vi "Process.vi"(8 "error in":errorcluster, 11 "Example Instrument UI":refnum<class "Instrument.PPMS2 UI.lvclass">) -> (0 "error out":errorcluster, 3 "Example Instrument UI out":refnum<class "Instrument.PPMS2 UI.lvclass">)   [LabVIEW 2016, in "Instrument.PPMS2 UI.lvclass"]
doc: "---------------------------------------------------------------\nJKI State Machine Objects™\nhttp://jki.net/state-machine-objects/\nCopyright (C) 2005-2015, JKI <info@jki.net>\nALL RIGHTS RESERVEDJKI State Machine Objects (SMO) 1.0.0.5\nJKI - JKI\nCopyright (c) 2016, JKI"
uses:
  Instrument.PPMS2 UI.lvclass
  C:/Program Files (x86)/National Instruments/LabVIEW 2016/vi.lib/JKI/JKI SMO/SMO/SMO.lvclass
  C:/Program Files (x86)/National Instruments/LabVIEW 2016/vi.lib/JKI/JKI SMO/SMO.UI/SMO.UI.lvclass
  instrument.PPMS2/Typedefs/Magnet Status--PPMS2--ring.ctl
  instrument.PPMS2/Typedefs/Temperature Status--PPMS2--ring.ctl
  <vilib>/JKI/JKI SMO/SMO/Typedefs/Parent Call--Enum.ctl
  <userlib>/LevyLab/Levylab Instruments/SMOs/RemoteControl.STM/RemoteControl.STM.lvclass
  Instrument.PPMS2 UI.lvclass/Instrument.PPMS2 UI.ctl
  instrument.PPMS2/Typedefs/getAll--PPMS2--cluster.ctl
  <vilib>/JKI/JKI SMO/SMO.UI/SMO.UI.lvclass
  <userlib>/LevyLab/Levylab Instruments/SMOs/Instrument/Instrument.lvclass
  <vilib>/JKI/JKI SMO/SMO/SMO.lvclass
  instrument.PPMS2/instrument.PPMS2.lvclass
panel:
  in  "Angle":bool
  in  "Field":bool
  in  "Temperature":bool
  in  "Target Angle (°)":dbl=-0.00643419474363327 format="%_3g"
  in  "Target Field (Oe)":dbl=-0.00643419474363327 format="%_3g"
  in  "Target Temperature (K)":dbl=305.0156 format="%#_5g"
  out "Temperature Status":T1 items=["TemperatureUnknown"=0, "Stable"=1, "Tracking"=2, "Near"=5, "Chasing"=6, "Filling"=7, "Standby"=10, "Disabled"=13, "ImpedanceNotFunction"=14, "TempFailure"=15]
  out "Field Status":T2=1 items=["MagnetUnknown"=0, "StablePersistent"=1, "WarmingSwitch"=2, "CoolingSwitch"=3, "StableDriven"=4, "Iterating"=5, "Charging"=6, "Discharging"=7, "CurrentError"=8, "MagnetFailure"=15]
  out "Helium Level (%)":dbl=86.7
  out "Position (°)":dbl=90.002
  out "Field (Oe)":dbl=-0.00643419474363327 format="%_3g"
  out "Temperature(K)":dbl=305.0156 format="%#_5g"
  in  "update time (ms)":u32=200
  in  "STOP":bool
  # "PPMS 2 Monitor"
  # "SMO UI Template"
  # "For instructions on how to use the JKI State Machine Objects, examples and video tutorials, visit:\nhttp://jki.net/state-machine-objects/\n\nJKI State Machine Objects™\nhttp://jki.net/state-machine-objects/\nCopyright (C) 2005-2015, JKI <info@jki.net>\nALL RIGHTS RESERVED"
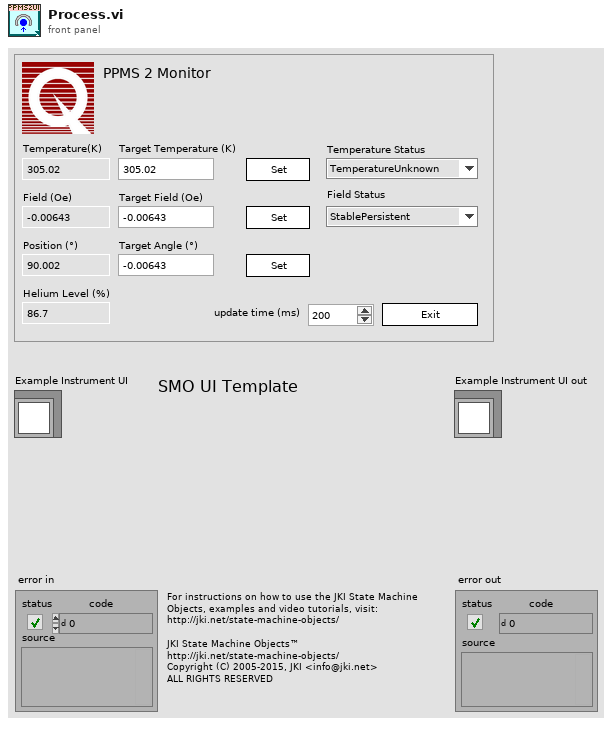
[diagram p1: front panel]
types:
  T1 = typedef "instrument.PPMS2.lvclass/Temperature Status--PPMS2--ring.ctl" = i32
  T2 = typedef "instrument.PPMS2.lvclass/Magnet Status--PPMS2--ring.ctl" = i32
  T3 = typedef "SMO.lvclass/Parent Call--Enum.ctl" = enum16{"Allows parent to run", "Does not request parent to run"}
  T4 = enum32{"invalid app kind", "Development System", "Run Time System", "Student Edition", "Embedded LabVIEW", "Evaluation", "Custom"}
  T5 = enum32{"Invalid", "Standard", "Closed", "Hidden", "Minimized", "Maximized"}
  T6 = typedef "instrument.PPMS2.lvclass/getAll--PPMS2--cluster.ctl" = cluster{"PPMS 2 Helium Level":dbl, "PPMS 2 Temperature":dbl, "PPMS 2 Temperature Status":T1, "PPMS 2 Magnetic Field":dbl, "PPMS 2 Magnet Status":T2, "PPMS 2 Position":dbl}
  T7 = cluster{"Core":cluster{"Current VI Reference":refnum<vi>, "Close Panel on Exit?":bool, "error":errorcluster}, "Self Reference":refnum<class "Instrument.PPMS2 UI.lvclass">, "Instrument":refnum<class "Instrument.lvclass">, "RC.STM":refnum<class "RemoteControl.STM.lvclass">, "getAll":variant, "getDisplay":variant, "config":variant}
  T8 = cluster{"Current VI Reference":refnum<vi>, "Close Panel on Exit?":bool, "error":errorcluster}
  T9 = typedef "SMO.lvclass/Protected Events.ctl" = cluster{"StopProcesses":refnum<user-event>, "AbortProcesses":refnum<user-event>, "Config Changed":refnum<user-event>, "Dependency":refnum<user-event>}
  T10 = typedef "Instrument.lvclass/PublicEvents--Cluster.ctl" = cluster{"MessageFromProcess":refnum<user-event>}
  T11 = typedef "Instrument.lvclass/Configuration--Cluster.ctl" = cluster{"Hardware":cluster{"Address":string, "Type":string, "COM Type":string}, "SMO":cluster{"VI Address":string, "Port":i32}, "DSC":cluster{"Process Name":string}}
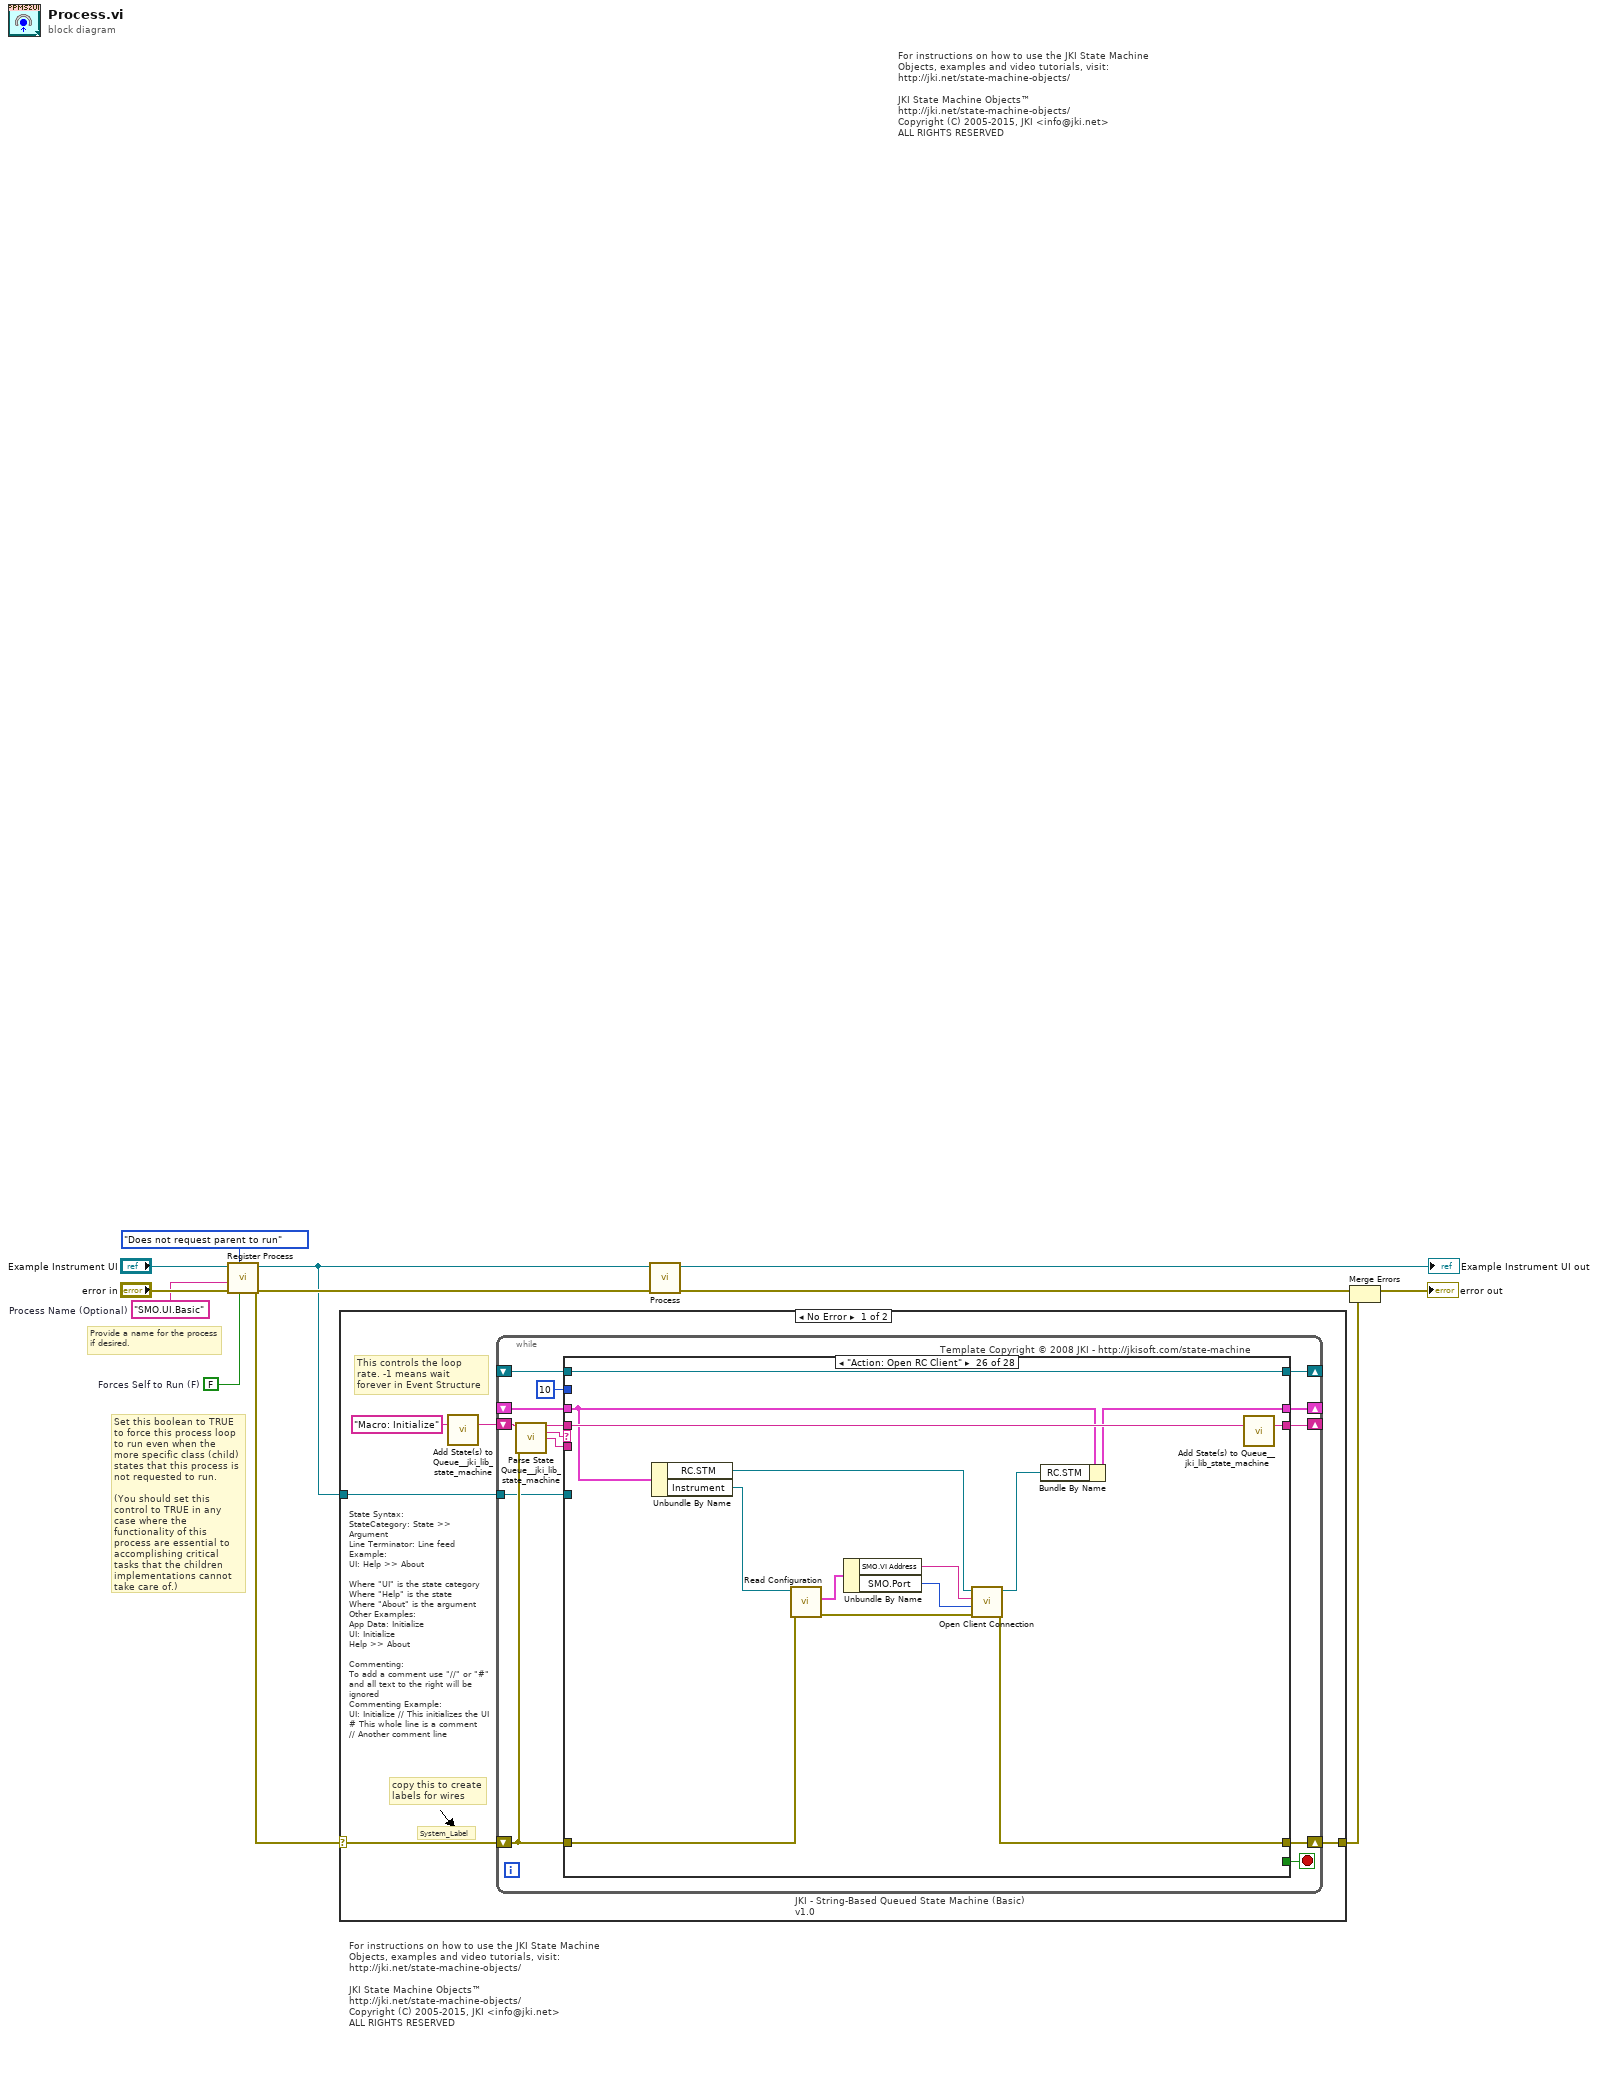
[diagram p0: block diagram]
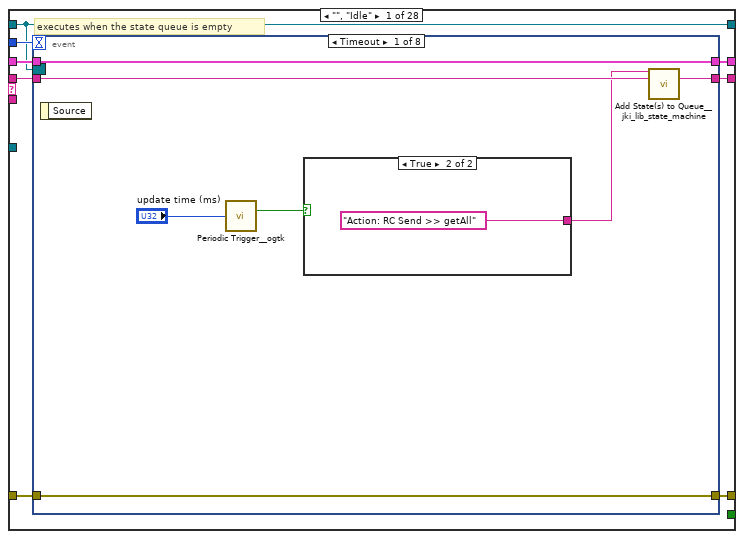
[diagram p2: hidden frame]
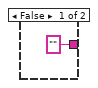
[diagram p3: hidden frame]
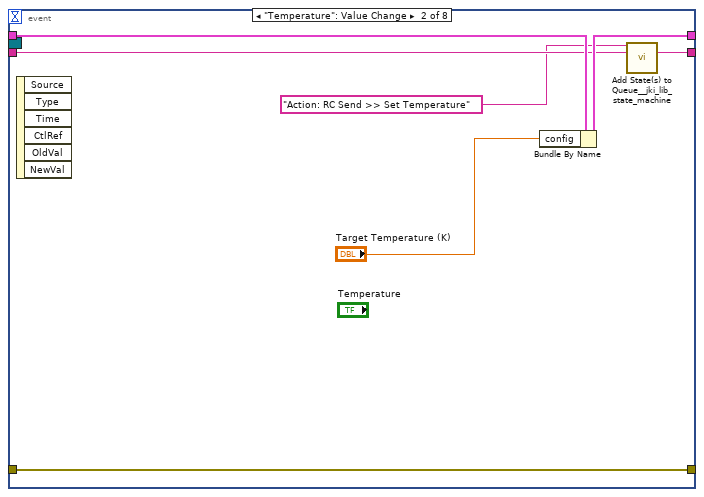
[diagram p4: hidden frame]
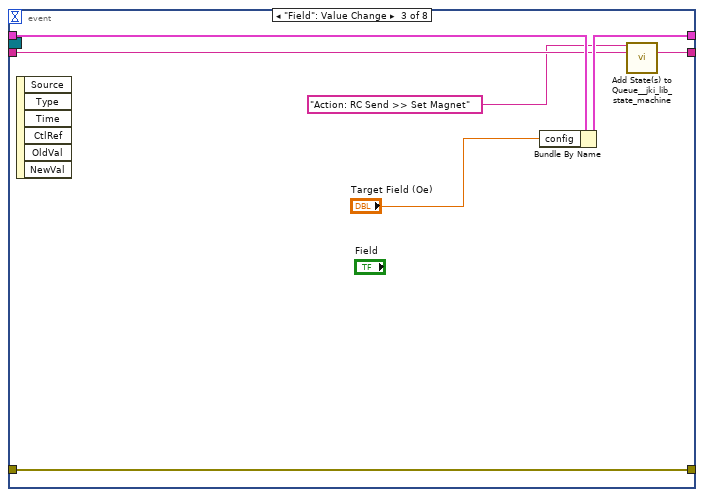
[diagram p5: hidden frame]
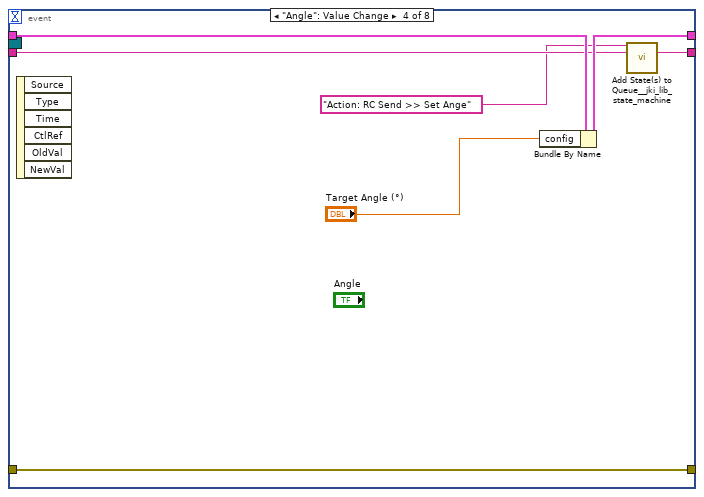
[diagram p6: hidden frame]
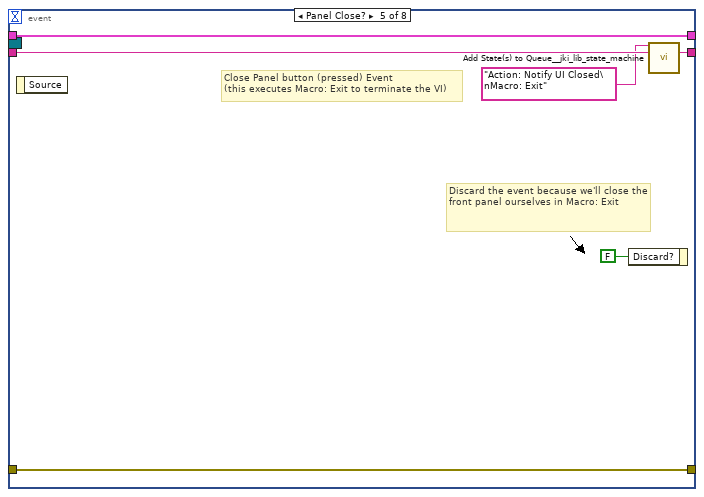
[diagram p7: hidden frame]
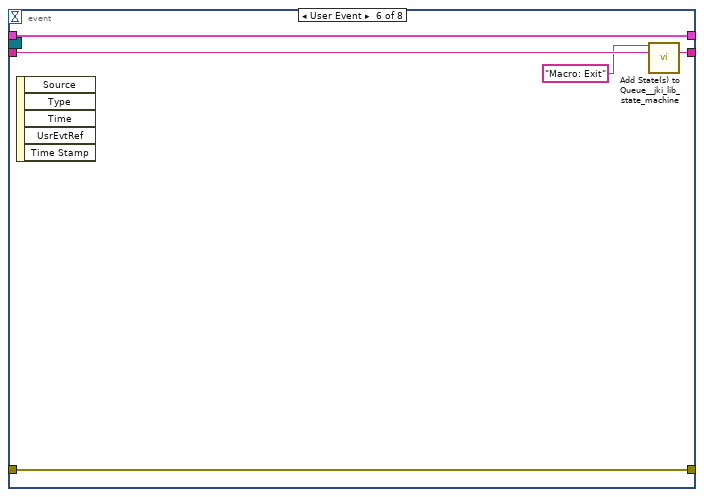
[diagram p8: hidden frame]
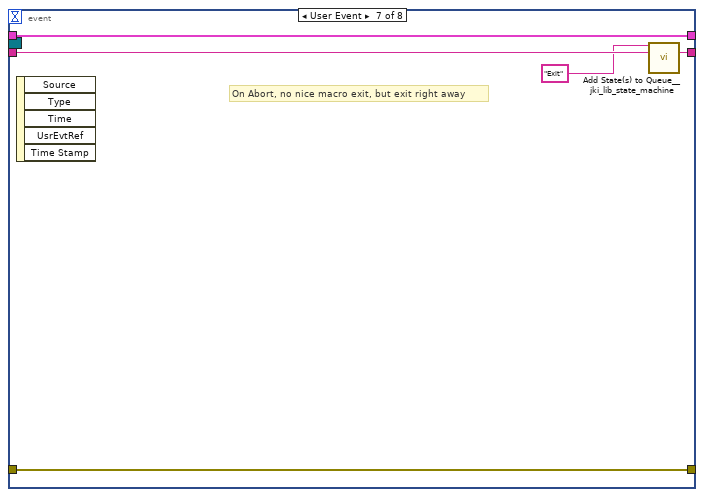
[diagram p9: hidden frame]
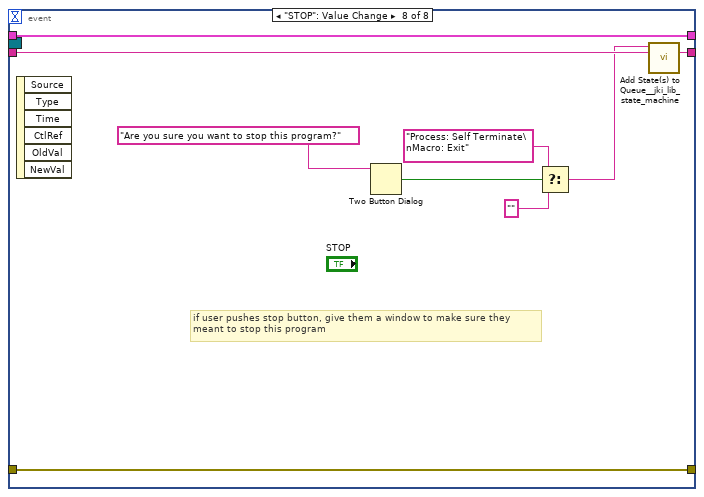
[diagram p10: hidden frame]
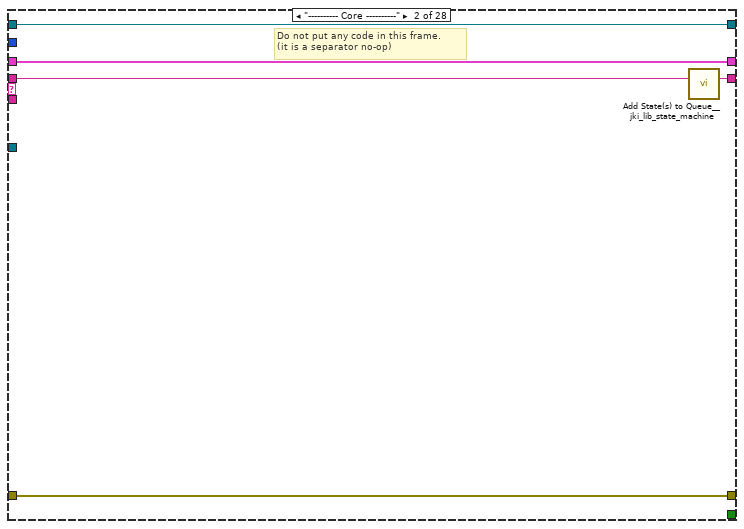
[diagram p11: hidden frame]
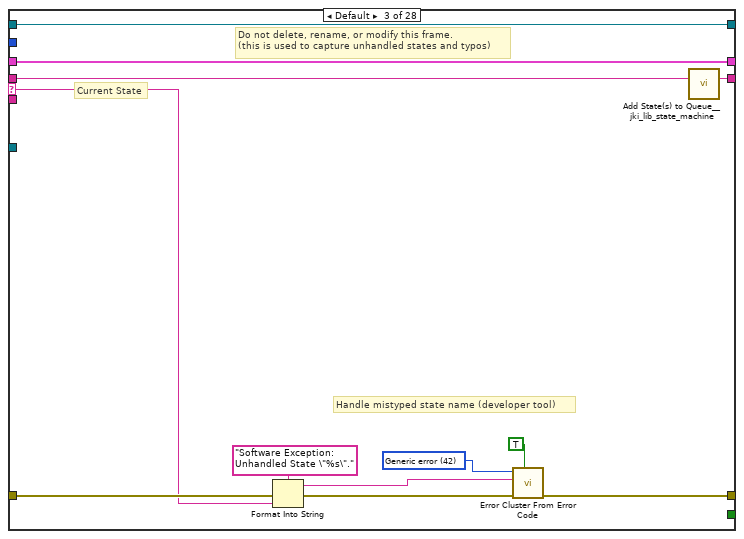
[diagram p12: hidden frame]
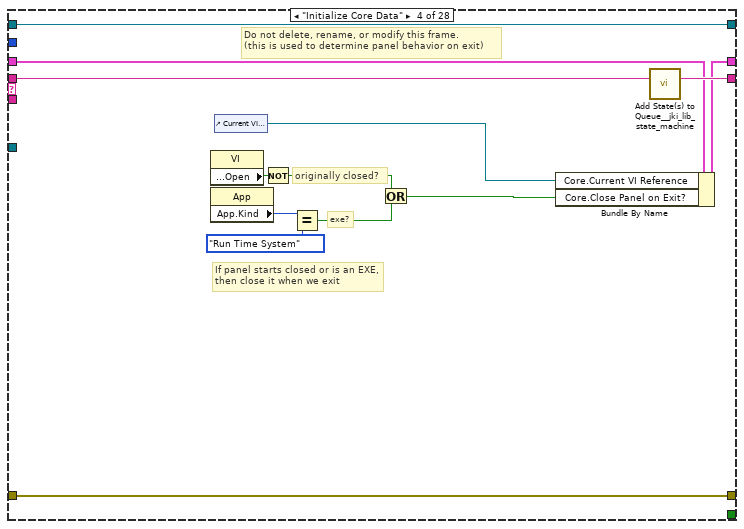
[diagram p13: hidden frame]
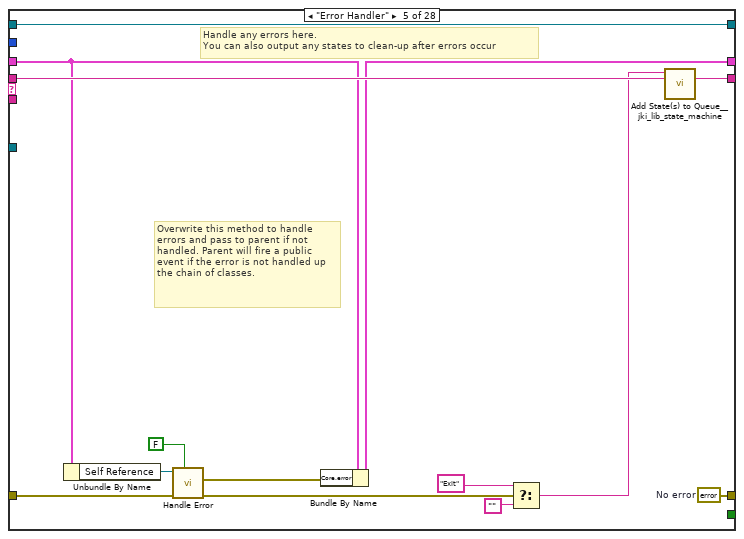
[diagram p14: hidden frame]
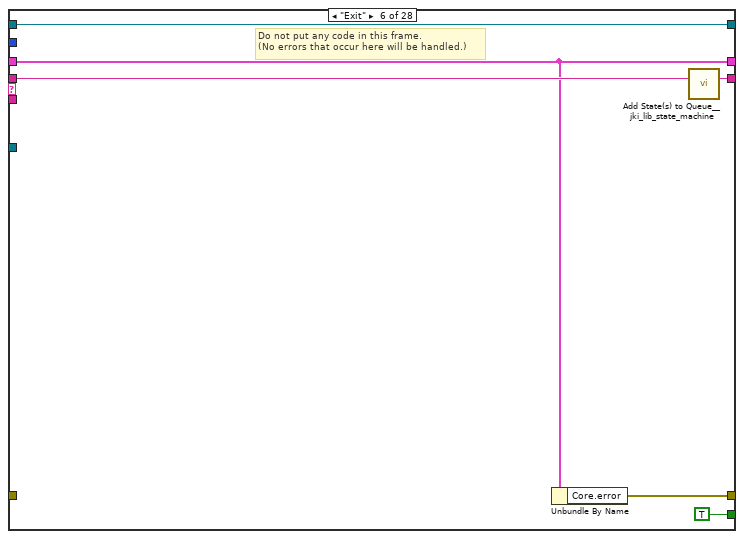
[diagram p15: hidden frame]
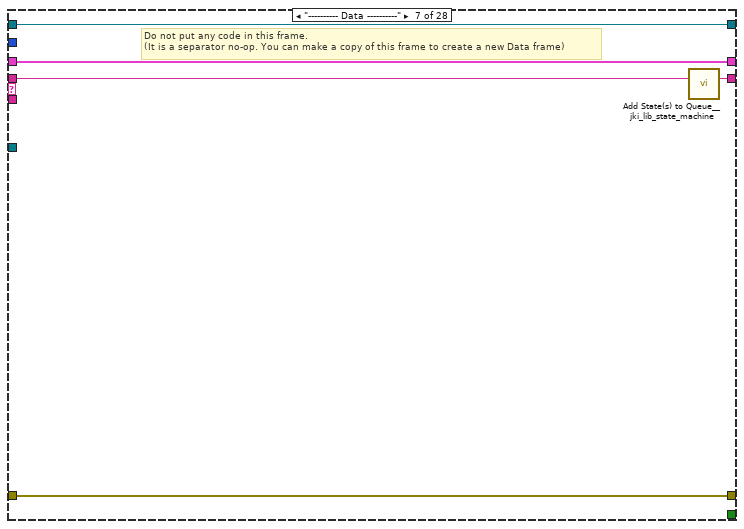
[diagram p16: hidden frame]
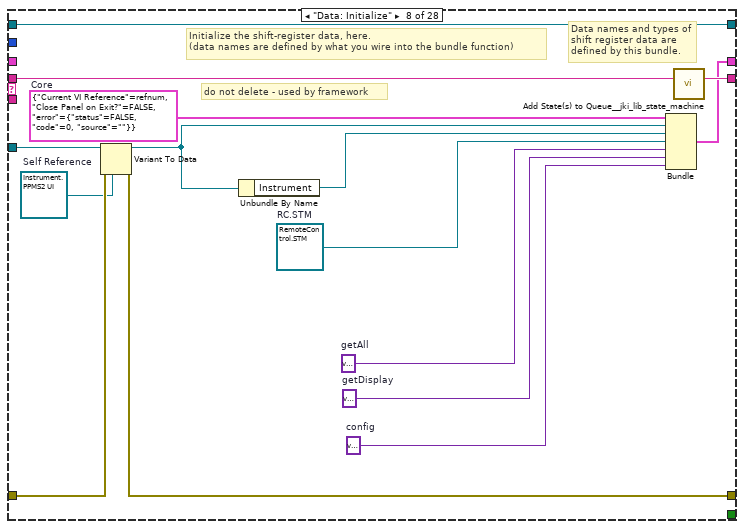
[diagram p17: hidden frame]
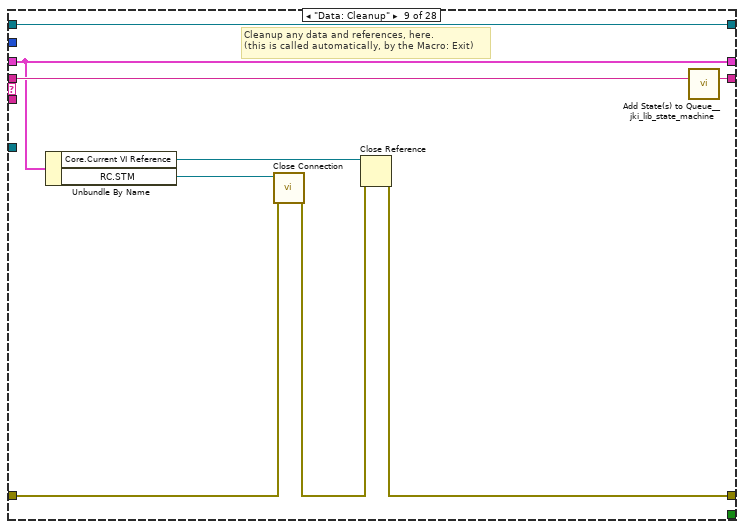
[diagram p18: hidden frame]
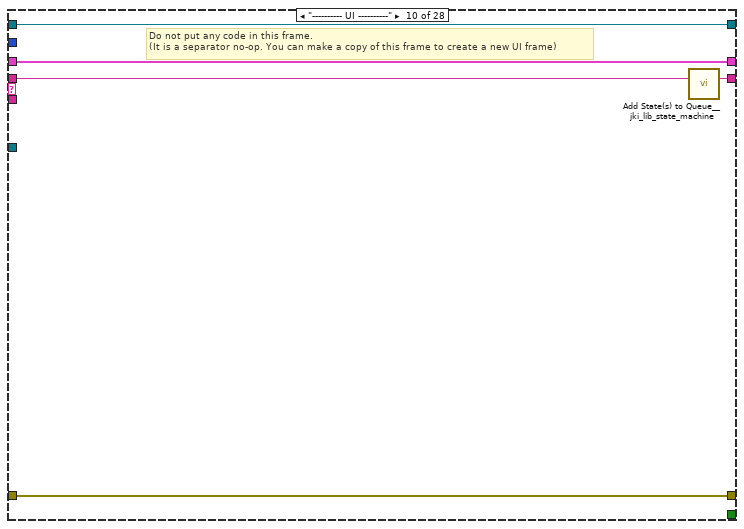
[diagram p19: hidden frame]
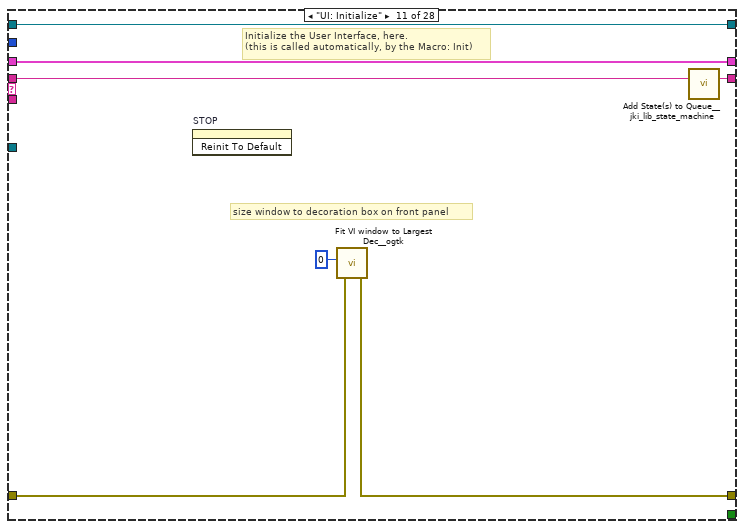
[diagram p20: hidden frame]
diagram:
  w2 = FALSE  # Forces Self to Run (F)
  w1 = "SMO.UI.Basic"  # Process Name (Optional)
  # "For instructions on how to use the JKI State Machine Objects, examples and video tutorials, visit:\nhttp://jki.net/state-machine-objects/\n\nJKI State Machine Objects™\nhttp://jki.net/state-machine-objects/\nCopyright (C) 2005-2015, JKI <info@jki.net>\nALL RIGHTS RESERVED"
  # "Provide a name for the process\nif desired."
  # "Set this boolean to TRUE to force this process loop to run even when the more specific class (child) states that this process is not requested to run.\n\n(You should set this control to TRUE in any case where the functionality of this process are essential to accomplishing critical tasks that the children implementations cannot take care of.)"
  # "For instructions on how to use the JKI State Machine Objects, examples and video tutorials, visit:\nhttp://jki.net/state-machine-objects/\n\nJKI State Machine Objects™\nhttp://jki.net/state-machine-objects/\nCopyright (C) 2005-2015, JKI <info@jki.net>\nALL RIGHTS RESERVED"
  n1 = call <vilib>:"Register Process.vi"("Forces Self to Run (F)"=w2, "Parent Call"=Parent_Call--Enum."Does not request parent to run", "error in (no error)"="error in", "Process Name (optional)"=w1, "SMO"="Example Instrument UI") -> ("error out"=w8:errorcluster, "SMO out"=w7:refnum<class "Instrument.PPMS2 UI.lvclass">)  [unwired: 5 in]
  n2 = case shown="No Error" w8 {
    selector: w8 -> [w13 w389]
    tunnel: w7 -> [w14 _]
    tunnel: [w12 w389] -> w4
    frame No Error {
      # "State Syntax:\nStateCategory: State >> Argument\nLine Terminator: Line feed\nExample:\nUI: Help >> About\n\nWhere \"UI\" is the state category\nWhere \"Help\" is the state\nWhere \"About\" is the argument\nOther Examples:\nApp Data: Initialize\nUI: Initialize\nHelp >> About\n\nCommenting:\nTo add a comment use \"//\" or \"#\" and all text to the right will be ignored\nCommenting Example:\nUI: Initialize // This initializes the UI\n# This whole line is a comment\n// Another comment line"
      # "copy this to create labels for wires"
      # "This controls the loop rate. -1 means wait forever in Event Structure"
      # "System_Label"
      n3 = call <vilib>:"Add State(s) to Queue__jki_lib_state_machine.vi"("State(s) in (\"\")"="Macro: Initialize") -> ("States Out"=w16:string)  [unwired: 14 in]
      n4 = while "JKI - String-Based Queued State Machine (Basic) v1.0" {
        shift-right: [w23] -> _
        shift-left: _ -> [w22]
        shift-right: [w26] -> w12
        shift-left: w13 -> [w20]
        shift-right: [w25] -> _
        shift-left: w16 -> [w27]
        tunnel: w14 -> [w19]
        shift-right: [w18] -> _
        shift-left: _ -> [w17]
        stop <- w24 stop-if-true
        # "Template Copyright © 2008 JKI - http://jkisoft.com/state-machine"
        n5 = call <vilib>:"Parse State Queue__jki_lib_state_machine.vi"("State Queue"=w27, "Error In (no error)"=w20) -> ("Remaining States"=w29:string, "Current State"=w30:string, "Arguments"=w28:string)  [unwired: 11 in]
        n6 = case shown="\"Action: Open RC Client\"" w30 {
          selector: w30 -> [_ _ w100 _ _ _ _ _ _ _ _ _ _ _ _ _ _ _ _ _ _ _ _ _ _ _ _ _]
          tunnel: w29 -> [w38 w98 w104 w123 w137 w143 w148 w163 w172 w177 w184 w191 w207 w239 w248 w262 w267 w278 w285 w290 w303 w309 w316 w323 w338 w352 w369 w388]
          tunnel: w28 -> [_ _ _ _ _ _ _ _ _ _ _ w185 w201 _ _ _ _ _ _ _ _ _ _ _ _ _ w355 w380]
          tunnel: w22 -> [w36 w95 w102 w114 w125 w139 w145 _ w168 w174 w182 w189 w203 w236 w244 w253 w264 w275 w280 w287 w301 w307 w312 w319 w335 w343 w366 w385]
          tunnel: [w35 w96 w106 w120 w130 w138 w146 w159 w169 w175 w179 w186 w204 w237 w246 w260 w265 w269 w281 w288 w296 w304 w313 w317 w333 w340 w359 w383] -> w26
          tunnel: w20 -> [w34 w96 w105 w120 w126 _ w146 w160 w165 w175 w180 w187 w205 w237 w246 w260 w265 w270 w282 w288 w298 w305 w313 w318 w334 w341 w362 w381]
          tunnel: [w37 w97 w103 w122 w136 w142 w147 w162 w171 w176 w183 w190 w206 w238 w247 w261 w266 w277 w284 w289 w302 w308 w315 w322 w337 w351 w368 w387] -> w25
          tunnel: [_ _ _ _ _ TRUE _ _ _ _ _ _ _ _ _ _ _ _ _ _ _ _ _ _ _ _ _ _] -> w24
          tunnel: [w33 w95 w102 w121 w128 w139 w145 w161 w168 w174 w182 w189 w203 w236 w244 w253 w264 w275 w280 w287 w301 w307 w311 w319 w335 w342 w365 w385] -> w23
          tunnel: 10 ("Timeout") -> [w32 _ _ _ _ _ _ _ _ _ _ _ _ _ _ _ _ _ _ _ _ _ _ _ _ _ _ _]
          tunnel: w19 -> [_ _ _ _ _ _ _ w157 _ _ _ _ _ _ _ _ _ _ _ _ _ _ _ _ _ _ _ _]
          tunnel: [w31 w94 w99 w111 w135 w140 w144 w156 w167 w173 w181 w188 w200 w235 w245 w254 w263 w276 w283 w286 w300 w306 w314 w321 w336 w350 w367 w386] -> w18
          tunnel: w17 -> [w31 w94 w99 w111 w135 w140 w144 w156 w167 w173 w181 w188 w200 w235 w245 w254 w263 w276 w283 w286 _ w306 w314 w321 w336 w350 w367 w386]
          frame "", "Idle" {
            # "executes when the state queue is empty"
            n7 = event shown="[0] Timeout" {
              selector: w31 -> [_ _ _ _ _ _ _ _]
              dyn-events: _ -> [_ _ _ _ _ _ _ _]
              timeout: w32 -> [_ _ _ _ _ _ _ _]
              tunnel: w38 -> [w45 w50 w57 w64 w74 w79 w84 w93]
              tunnel: [w44 w53 w60 w67 w73 w78 w83 w92] -> w37
              tunnel: w36 -> [w42 w52 w59 w66 w70 w76 w81 w90]
              tunnel: [w43 w54 w61 w68 w69 w77 w82 w91] -> w35
              tunnel: w34 -> [w43 w54 w61 w68 w69 w77 w82 w91]
              tunnel: [w42 w51 w58 w65 w70 w76 w81 w90] -> w33
              event Timeout {
                n8 = event-data() -> ()  [unwired: 1 in, 1 out]
                n9 = call <userlib>:"Periodic Trigger__ogtk.vi"("time (ms)"="update time (ms)") -> ("Triggered"=w41:bool)  [unwired: 12 in, 2 out]
                n10 = case shown="True" w41 {
                  tunnel: ["" "Action: RC Send >> getAll"] -> w39
                  frame False {
                  }
                  frame True {
                  }
                }
                n11 = call <vilib>:"Add State(s) to Queue__jki_lib_state_machine.vi"("State(s) in Front (\"\")"=w39, "State(s) in (\"\")"=w45) -> ("States Out"=w44:string)  [unwired: 13 in]
              }
              event "Temperature": Value Change {
                n12 = event-data() -> ()  [unwired: 1 in, 6 out]
                n13 = Bundle By Name(cluster=w52, "config"="Target Temperature (K)") -> (w51:T7)
                n14 = call <vilib>:"Add State(s) to Queue__jki_lib_state_machine.vi"("State(s) in Front (\"\")"="Action: RC Send >> Set Temperature" ("State(s) in Front (\"\")"), "State(s) in (\"\")"=w50) -> ("States Out"=w53:string)  [unwired: 13 in]
              }
              event "Field": Value Change {
                n15 = event-data() -> ()  [unwired: 1 in, 6 out]
                n16 = Bundle By Name(cluster=w59, "config"="Target Field (Oe)") -> (w58:T7)
                n17 = call <vilib>:"Add State(s) to Queue__jki_lib_state_machine.vi"("State(s) in Front (\"\")"="Action: RC Send >> Set Magnet" ("State(s) in Front (\"\")"), "State(s) in (\"\")"=w57) -> ("States Out"=w60:string)  [unwired: 13 in]
              }
              event "Angle": Value Change {
                n18 = event-data() -> ()  [unwired: 1 in, 6 out]
                n19 = Bundle By Name(cluster=w66, "config"="Target Angle (°)") -> (w65:T7)
                n20 = call <vilib>:"Add State(s) to Queue__jki_lib_state_machine.vi"("State(s) in Front (\"\")"="Action: RC Send >> Set Ange" ("State(s) in Front (\"\")"), "State(s) in (\"\")"=w64) -> ("States Out"=w67:string)  [unwired: 13 in]
              }
              event Panel Close? {
                # "Discard the event because we'll close the front panel ourselves in Macro: Exit"
                # "Close Panel button (pressed) Event\n(this executes Macro: Exit to terminate the VI)"
                n21 = event-data() -> ()  [unwired: 1 in, 1 out]
                n22 = event-data("Discard?"=FALSE) -> ()  [unwired: 1 in, 1 out]
                n23 = call <vilib>:"Add State(s) to Queue__jki_lib_state_machine.vi"("State(s) in Front (\"\")"="Action: Notify UI Closed\nMacro: Exit", "State(s) in (\"\")"=w74) -> ("States Out"=w73:string)  [unwired: 13 in]
              }
              event User Event {
                n24 = event-data() -> ()  [unwired: 1 in, 5 out]
                n25 = call <vilib>:"Add State(s) to Queue__jki_lib_state_machine.vi"("State(s) in Front (\"\")"="Macro: Exit", "State(s) in (\"\")"=w79) -> ("States Out"=w78:string)  [unwired: 13 in]
              }
              event User Event {
                # "On Abort, no nice macro exit, but exit right away"
                n26 = event-data() -> ()  [unwired: 1 in, 5 out]
                n27 = call <vilib>:"Add State(s) to Queue__jki_lib_state_machine.vi"("State(s) in Front (\"\")"="Exit", "State(s) in (\"\")"=w84) -> ("States Out"=w83:string)  [unwired: 13 in]
              }
              event "STOP": Value Change {
                # "if user pushes stop button, give them a window to make sure they\nmeant to stop this program"
                n28 = event-data() -> ()  [unwired: 1 in, 6 out]
                n29 = Two Button Dialog(message="Are you sure you want to stop this program?") -> (T button?=w89:bool)  [unwired: 2 in]
                n30 = Select(t="Process: Self Terminate\nMacro: Exit", s=w89, f="") -> (s? t:f=w85:string)
                n31 = call <vilib>:"Add State(s) to Queue__jki_lib_state_machine.vi"("State(s) in Front (\"\")"=w85, "State(s) in (\"\")"=w93) -> ("States Out"=w92:string)  [unwired: 13 in]
              }
            }
          }
          frame "---------- Core ----------" {
            # "Do not put any code in this frame.\n(it is a separator no-op)"
            n32 = call <vilib>:"Add State(s) to Queue__jki_lib_state_machine.vi"("State(s) in (\"\")"=w98) -> ("States Out"=w97:string)  [unwired: 14 in]
          }
          frame Default {
            w109 = 42 items=["No error", "Argument error", "Memory is full", "Out of zone", "End of file", "File already open", "Generic file I/O error", "File not found", "File permission error", "Disk is full", "Duplicate path", "Too many files open", "System feature not enabled", "Resource file not found", "Cannot add resource", "Resource not found", "Image not found", "Image memory error", "Pen does not exist", "Config type invalid", "Config token not found", "Config parse error", "Config memory error", "Bad external code format", "Bad external code offset", "External code not present", "Null window", "Destroy window error", "Null menu", "Print aborted", "Bad print record", "Print driver error", "Windows error during printing", "Memory error during printing", "Print dialog error", "Generic print error", "Invalid device refnum", "Device not found", "Device parameter error", "Device unit error", "Cannot open device", "Device call aborted", "Generic error", "Cancelled by user", "Object ID too low", "Object ID too high", "Object not in heap", "Unknown heap", "Unknown object (invalid DefProc)", "Unknown object (DefProc not in table)", "Message out of range", "Invalid (null) method", "Unknown message", "Manager call not supported", "Bad address", "Network operation in progress", "Network operation timed out", "Connection is busy", "Network attribute not supported", "Network error", "Address in use", "System out of memory", "Connection aborted", "Connection refused", "Not connected", "Already connected", "Connection closed", "Initialization error (interapplication manager)", "Bad occurrence", "Wait on unbound occurrence handler", "Occurrence queue overflow", "Datalog type conflict", "Unused", "Unrecognized type (interapplication manager)", "Memory corrupt", "Failed to make temporary DLL", "Old CIN version", "Drag socket not found", "Failed to load drop-object", "Failed to register OLE object", "Failed to release OLE object", "Format specifier type mismatch", "Unknown format specifier", "Too few format specifiers", "Too many format specifiers", "Scan failed", "Newer CIN version", "Error converting to variant", "Runtime menu error", "Password tampered", "Variant attribute not found", "Incompatible variant data type", "Event data is not available", "Event Store is not present", "Occurrence is not found", "Event Queue is not created", "Event info is not available", "Refnum passed is NULL", "Error retrieving Class GUID", "Error retrieving CoClass GUID", "Error retrieving TypeLib GUID.", "Bad built application magic bytes.", "Specific driver is different from the specific driver associated with the Logical Name.", "There is no session opened to the class driver.", "Max Error", "MAX - Error with config objects", "MAX - Error loading configuration", "MAX - Group not supported"]
            # "Current State"
            # "Do not delete, rename, or modify this frame.\n(this is used to capture unhandled states and typos)"
            # "Handle mistyped state name (developer tool)"
            n33 = Format Into String(format string="Software Exception: Unhandled State \"%s\"." ("message"), error in=w105, w100) -> (resulting string=w108:string, error out=w107:errorcluster)  [unwired: 1 in]
            n34 = call <vilib>:"Error Cluster From Error Code.vi"("show call chain? (False)"=TRUE, "error in (no error)"=w107, "error message (\"\")"=w108, "error code (0)"=w109) -> ("error out"=w106:errorcluster)  [unwired: 5 in]
            n35 = call <vilib>:"Add State(s) to Queue__jki_lib_state_machine.vi"("State(s) in (\"\")"=w104) -> ("States Out"=w103:string)  [unwired: 14 in]
          }
          frame "Initialize Core Data" {
            # "Do not delete, rename, or modify this frame.\n(this is used to determine panel behavior on exit)"
            # "originally closed?"
            # "exe?"
            # "If panel starts closed or is an EXE, then close it when we exit"
            n36 = property class="VI"() -> ("Front Panel.Open"=w119:bool)  [unwired: 2 in, 2 out]
            n37 = property class="App"() -> ("App.Kind"=w118:T4)  [unwired: 2 in, 2 out]
            n38 = control-ref of="Current VI Reference"() -> (w112:refnum<vi>)
            n39 = Not(x=w119) -> (.not. x?=w116:bool)
            n40 = Equal?(x=w118, y=T4."Run Time System" ("Application:Kind")) -> (x = y?=w115:bool)
            n41 = Or(x=w116, y=w115) -> (x .or. y?=w113:bool)
            n42 = Bundle By Name(cluster=w114, "Core.Current VI Reference"=w112, "Core.Close Panel on Exit?"=w113) -> (w121:T7)
            n43 = call <vilib>:"Add State(s) to Queue__jki_lib_state_machine.vi"("State(s) in (\"\")"=w123) -> ("States Out"=w122:string)  [unwired: 14 in]
          }
          frame "Error Handler" {
            w130 = errorcluster {"status"=FALSE, "code"=0, "source"=""}  # No error
            # "Overwrite this method to handle errors and pass to parent if not handled. Parent will fire a public event if the error is not handled up the chain of classes."
            # "Handle any errors here.\nYou can also output any states to clean-up after errors occur"
            n44 = Unbundle By Name(w125) -> ("Self Reference"=w134:refnum<class "Instrument.PPMS2 UI.lvclass">)
            n45 = call-dynamic "Handle Error.vi"("Stop on Unhandled Error (T)"=FALSE, "error in"=w126, "SMO"=w134) -> ("handling error"=w124:errorcluster, "Unhandled error"=w129:errorcluster)  [unwired: 6 in, 1 out]
            n46 = Bundle By Name(cluster=w125, "Core.error"=w129) -> (w128:T7)
            n47 = Select(t="Exit", s=w124, f="") -> (s? t:f=w131:string)
            n48 = call <vilib>:"Add State(s) to Queue__jki_lib_state_machine.vi"("State(s) in Front (\"\")"=w131, "State(s) in (\"\")"=w137) -> ("States Out"=w136:string)  [unwired: 13 in]
          }
          frame "Exit" {
            # "Do not put any code in this frame.\n(No errors that occur here will be handled.)"
            n49 = Unbundle By Name(w139) -> ("Core.error"=w138:errorcluster)
            n50 = call <vilib>:"Add State(s) to Queue__jki_lib_state_machine.vi"("State(s) in (\"\")"=w143) -> ("States Out"=w142:string)  [unwired: 14 in]
          }
          frame "---------- Data ----------" {
            # "Do not put any code in this frame.\n(It is a separator no-op. You can make a copy of this frame to create a new Data frame)"
            n51 = call <vilib>:"Add State(s) to Queue__jki_lib_state_machine.vi"("State(s) in (\"\")"=w148) -> ("States Out"=w147:string)  [unwired: 14 in]
          }
          frame "Data: Initialize" {
            w149 = refnum<class "RemoteControl.STM.lvclass"> refnum  # RC.STM
            w151 = variant  # config
            w152 = variant  # getDisplay
            w153 = variant  # getAll
            w155 = T8 {"Current VI Reference"=refnum, "Close Panel on Exit?"=FALSE, "error"={"status"=FALSE, "code"=0, "source"=""}}  # Core
            w158 = refnum<class "Instrument.PPMS2 UI.lvclass"> refnum  # Self Reference
            # "do not delete - used by framework"
            # "Data names and types of shift register data are defined by this bundle."
            # "Initialize the shift-register data, here.\n(data names are defined by what you wire into the bundle function)"
            n52 = Variant To Data(error in=w160, type=w158, Variant=w157) -> (data=w154:refnum<class "Instrument.PPMS2 UI.lvclass">, error out=w159:errorcluster)
            n53 = Unbundle By Name(w154) -> ("Instrument"=w150:refnum<class "Instrument.lvclass">)
            n54 = Bundle("Core"=w155, "Self Reference"=w154, "Instrument"=w150, "RC.STM"=w149, "getAll"=w153, "getDisplay"=w152, "config"=w151) -> (w161:T7)  [unwired: 1 in]
            n55 = call <vilib>:"Add State(s) to Queue__jki_lib_state_machine.vi"("State(s) in (\"\")"=w163) -> ("States Out"=w162:string)  [unwired: 14 in]
          }
          frame "Data: Cleanup" {
            # "Cleanup any data and references, here.\n(this is called automatically, by the Macro: Exit)"
            n56 = Unbundle By Name(w168) -> ("Core.Current VI Reference"=w170:refnum<vi>, "RC.STM"=w166:refnum<class "RemoteControl.STM.lvclass">)
            n57 = call-dynamic "Close Connection.vi"("error in (no error)"=w165, "RemoteControl.STM in"=w166) -> ("error out"=w164:errorcluster)  [unwired: 8 in, 1 out]
            n58 = Close Reference(reference=w170, error in (no error)=w164) -> (error out=w169:errorcluster)
            n59 = call <vilib>:"Add State(s) to Queue__jki_lib_state_machine.vi"("State(s) in (\"\")"=w172) -> ("States Out"=w171:string)  [unwired: 14 in]
          }
          frame "---------- UI ----------" {
            # "Do not put any code in this frame.\n(It is a separator no-op. You can make a copy of this frame to create a new UI frame)"
            n60 = call <vilib>:"Add State(s) to Queue__jki_lib_state_machine.vi"("State(s) in (\"\")"=w177) -> ("States Out"=w176:string)  [unwired: 14 in]
          }
          frame "UI: Initialize" {
            # "size window to decoration box on front panel"
            # "Initialize the User Interface, here.\n(this is called automatically, by the Macro: Init)"
            n61 = invoke on="STOP" class="Bool (strict)" method="Reinit To Default"() -> ()  [unwired: 3 in, 3 out]
            n62 = call <userlib>:"Fit VI window to Largest Dec__ogtk.vi"("error in (no error)"=w180, "border spacing (2 px)"=0) -> ("error out"=w179:errorcluster)  [unwired: 4 in, 1 out]
            n63 = call <vilib>:"Add State(s) to Queue__jki_lib_state_machine.vi"("State(s) in (\"\")"=w184) -> ("States Out"=w183:string)  [unwired: 14 in]
          }
          frame "UI: Cursor Set" {
            # "Argument"
            # "Initialize the User Interface, here.\n(this is called automatically, by the Macro: Init)"
            n64 = disable-structure shown="Default" {
              disable-tunnel: w187 -> [w192 w195]
              disable-tunnel: [w192 w194] -> w186
              disable-tunnel: w185 -> [_ w193]
              frame condition #0 {
              }
              frame condition #1 (active) {
                n65 = case shown="\"Busy\"" w193 {
                  tunnel: w195 -> [w197 w199]
                  tunnel: [w196 w198] -> w194
                  frame "Idle", Default {
                    n66 = call <vilib>:"Unset Busy.vi"("error in (no error)"=w197) -> ("error out"=w196:errorcluster)  [unwired: 10 in]
                  }
                  frame "Busy" {
                    n67 = call <vilib>:"Set Busy.vi"("error in (no error)"=w199) -> ("error out"=w198:errorcluster)  [unwired: 9 in, 1 out]
                  }
                }
              }
            }
            n68 = call <vilib>:"Add State(s) to Queue__jki_lib_state_machine.vi"("State(s) in (\"\")"=w191) -> ("States Out"=w190:string)  [unwired: 14 in]
          }
          frame "UI: Front Panel State" {
            # "Argument"
            # "Set Front Panel Open or Closed\n(Usage: \"UI: Front Panel State >> Open|Close\")"
            n69 = Unbundle By Name(w203) -> ("Core.Current VI Reference"=w202:refnum<vi>)
            n70 = disable-structure shown="Default" {
              disable-tunnel: w205 -> [w211 w234]
              disable-tunnel: [w210 w234] -> w204
              disable-tunnel: w202 -> [w209 _]
              disable-tunnel: w201 -> [w208 _]
              frame condition #0 (active) {
                n71 = case shown="\"Close\"" w208 {
                  tunnel: w211 -> [w215 w228]
                  tunnel: [w217 w229] -> w210
                  tunnel: w209 -> [w216 w226]
                  frame "Open", Default {
                    n72 = property class="VI"(reference=w216, error in=w215) -> (reference out=w213:refnum<vi>, error out=w214:errorcluster, "FP.State"=w212:T5)
                    n73 = case shown="\"Closed\"" w212 {
                      tunnel: [w220 w223] -> w217
                      tunnel: w214 -> [w219 w223]
                      tunnel: w213 -> [w218 _]
                      frame "Closed" {
                        n74 = invoke class="VI" method="FP.Open"(reference=w218, error in=w219, "Activate"=TRUE, "State"=T5."Standard") -> (error out=w220:errorcluster)  [unwired: 1 in, 4 out]
                      }
                      frame Default {
                      }
                    }
                  }
                  frame "Close" {
                    n75 = property class="VI"(reference=w226, error in=w228) -> (reference out=w225:refnum<vi>, error out=w227:errorcluster, "FP.State"=w224:T5)
                    n76 = case shown="Default" w224 {
                      tunnel: [w230 w233] -> w229
                      tunnel: w227 -> [w230 w232]
                      tunnel: w225 -> [_ w231]
                      frame "Invalid", "Closed" {
                      }
                      frame Default {
                        n77 = invoke class="VI" method="FP.Close"(reference=w231, error in=w232) -> (error out=w233:errorcluster)  [unwired: 1 in, 2 out]
                      }
                    }
                  }
                }
              }
              frame condition #1 {
              }
            }
            n78 = call <vilib>:"Add State(s) to Queue__jki_lib_state_machine.vi"("State(s) in (\"\")"=w207) -> ("States Out"=w206:string)  [unwired: 14 in]
          }
          frame "---------- Macro ----------" {
            # "Do not put any code in this frame.\n(It is a separator no-op. You can make a copy of this frame to create a new Macro frame)"
            n79 = call <vilib>:"Add State(s) to Queue__jki_lib_state_machine.vi"("State(s) in (\"\")"=w239) -> ("States Out"=w238:string)  [unwired: 14 in]
          }
          frame "Macro: Initialize" {
            w242 = "UI: Initialize\nUI: Front Panel State >> Open\nAction: Open RC Client"  # UI: Initialize UI: Front Panel State >> Open Action: Open RC Client
            # "Initialization Macro\n(This is called once, when the VI starts)"
            n80 = call <vilib>:"Add State(s) to Queue__jki_lib_state_machine.vi"("State(s) in Front (\"\")"="Data: Initialize\nInitialize Core Data\nEvents: Register", "State(s) in (\"\")"="Process: Sync", "State(s) at Back (\"\")"=w242) -> ("States Out"=w241:string)  [unwired: 12 in]
            n81 = call <vilib>:"Add State(s) to Queue__jki_lib_state_machine.vi"("State(s) in Front (\"\")"=w241, "State(s) in (\"\")"=w248) -> ("States Out"=w247:string)  [unwired: 13 in]
          }
          frame "Macro: Exit" {
            # "Exit Macro\n(This is called once, when the VI exits)"
            n82 = Unbundle By Name(w253) -> ("Core.Close Panel on Exit?"=w259:bool)
            n83 = Select(t="UI: Front Panel State >> Close", s=w259, f="") -> (s? t:f=w256:string)
            n84 = call <vilib>:"Add State(s) to Queue__jki_lib_state_machine.vi"("State(s) in Front (\"\")"="Data: Cleanup\nEvents: Unregister", "State(s) in (\"\")"="Process: Sync", "State(s) at Back (\"\")"="Exit") -> ("States Out"=w250:string)  [unwired: 12 in]
            n85 = call <vilib>:"Add State(s) to Queue__jki_lib_state_machine.vi"("State(s) in (\"\")"=w256, "State(s) at Back (\"\")"=w250) -> ("States Out"=w255:string)  [unwired: 13 in]
            n86 = call <vilib>:"Add State(s) to Queue__jki_lib_state_machine.vi"("State(s) in Front (\"\")"=w255, "State(s) in (\"\")"=w262) -> ("States Out"=w261:string)  [unwired: 13 in]
          }
          frame "---------- Process ----------" {
            # "Template Separator\n(You can make a copy of, or modify, this frame)"
            n87 = call <vilib>:"Add State(s) to Queue__jki_lib_state_machine.vi"("State(s) in (\"\")"=w267) -> ("States Out"=w266:string)  [unwired: 14 in]
          }
          frame "Process: Sync" {
            n88 = Unbundle By Name(w275) -> ("Self Reference"=w271:refnum<class "Instrument.PPMS2 UI.lvclass">)
            n89 = call <vilib>:"WaitOnProcessSync.vi"("error in (no error)"=w270, "SMO"=w271) -> ("error out"=w269:errorcluster, "Don't run?"=w274:bool)  [unwired: 7 in, 1 out]
            n90 = Select(t="Data: Cleanup\nEvents: Unregister\nExit", s=w274, f="") -> (s? t:f=w268:string)
            n91 = call <vilib>:"Add State(s) to Queue__jki_lib_state_machine.vi"("State(s) in Front (\"\")"=w268, "State(s) in (\"\")"=w278) -> ("States Out"=w277:string)  [unwired: 13 in]
          }
          frame "Process: Self Terminate" {
            n92 = Unbundle By Name(w280) -> ("Self Reference"=w279:refnum<class "Instrument.PPMS2 UI.lvclass">)
            n93 = call <vilib>:"SelfTerminate.vi"("error in (no error)"=w282, "SMO in"=w279) -> ("error out"=w281:errorcluster)  [unwired: 8 in, 1 out]
            n94 = call <vilib>:"Add State(s) to Queue__jki_lib_state_machine.vi"("State(s) in (\"\")"=w285) -> ("States Out"=w284:string)  [unwired: 14 in]
          }
          frame "---------- Events ----------" {
            # "Template Separator\n(You can make a copy of, or modify, this frame)"
            n95 = call <vilib>:"Add State(s) to Queue__jki_lib_state_machine.vi"("State(s) in (\"\")"=w290) -> ("States Out"=w289:string)  [unwired: 14 in]
          }
          frame "Events: Register" {
            # "Expand to add\nmore events"
            # "Base Class Protected Events"
            n96 = Unbundle By Name(w301) -> ("Self Reference"=w294:refnum<class "Instrument.PPMS2 UI.lvclass">, "Instrument"=w293:refnum<class "Instrument.lvclass">)
            n97 = call <vilib>:"GetProtectedEvents.vi"("SMO"=w294) -> ("error out"=w295:errorcluster, "SMO Protected Events"=w299:T9)  [unwired: 8 in, 1 out]
            n98 = call <userlib>:"Instrument.GetPublicEvents.vi"("Instrument"=w293) -> ("error out"=w291:errorcluster, "Instrument Public Events"=w292:T10)  [unwired: 8 in, 1 out]
            n99 = register-events(w299, w292) -> (reference out=w300:refnum<event-registration>, error out=w297:errorcluster)  [unwired: 2 in]
            n100 = Merge Errors(w291, w298, w297, w295) -> (w296:errorcluster)
            n101 = call <vilib>:"Add State(s) to Queue__jki_lib_state_machine.vi"("State(s) in (\"\")"=w303) -> ("States Out"=w302:string)  [unwired: 14 in]
          }
          frame "Events: Unregister" {
            n102 = Unregister For Events(event registration refnum=w306, error in=w305) -> (error out=w304:errorcluster)
            n103 = call <vilib>:"Add State(s) to Queue__jki_lib_state_machine.vi"("State(s) in (\"\")"=w309) -> ("States Out"=w308:string)  [unwired: 14 in]
          }
          frame "---------- Action ----------" {
            n104 = Unbundle By Name(w312) -> ("Self Reference"=w310:refnum<class "Instrument.PPMS2 UI.lvclass">)
            n105 = Bundle By Name(cluster=w312, "Self Reference"=w310) -> (w311:T7)
            n106 = call <vilib>:"Add State(s) to Queue__jki_lib_state_machine.vi"("State(s) in (\"\")"=w316) -> ("States Out"=w315:string)  [unwired: 14 in]
          }
          frame "Action: Notify UI Closed" {
            # "Notify that the UI has been closed"
            n107 = Unbundle By Name(w319) -> ("Self Reference"=w320:refnum<class "Instrument.PPMS2 UI.lvclass">)
            n108 = call <vilib>:"Hide.vi"("error in (no error)"=w318, "SMO.UI"=w320) -> ("error out"=w317:errorcluster)  [unwired: 8 in, 1 out]
            n109 = call <vilib>:"Add State(s) to Queue__jki_lib_state_machine.vi"("State(s) in (\"\")"=w323) -> ("States Out"=w322:string)  [unwired: 14 in]
          }
          frame "Action: Update Front Panel All" {
            n110 = Unbundle By Name(w335) -> ("getAll"=w332:variant)
            n111 = Variant To Data(error in=w334, type=T6 {"PPMS 2 Helium Level"=0.0, "PPMS 2 Temperature"=0.0, "PPMS 2 Temperature Status"=0, "PPMS 2 Magnetic Field"=0.0, "PPMS 2 Magnet Status"=1, "PPMS 2 Position"=0.0} ("getAll"), Variant=w332) -> (data=w330:T6, error out=w333:errorcluster)
            n112 = Unbundle By Name(w330) -> ("PPMS 2 Helium Level"=→"Helium Level (%)":dbl, "PPMS 2 Temperature"=→"Temperature(K)":dbl, "PPMS 2 Temperature Status"=→"Temperature Status":T1, "PPMS 2 Magnetic Field"=→"Field (Oe)":dbl, "PPMS 2 Magnet Status"=→"Field Status":T2, "PPMS 2 Position"=→"Position (°)":dbl)
            n113 = call <vilib>:"Add State(s) to Queue__jki_lib_state_machine.vi"("State(s) in (\"\")"=w338) -> ("States Out"=w337:string)  [unwired: 14 in]
          }
          frame "Action: Open RC Client" {
            n114 = Unbundle By Name(w343) -> ("RC.STM"=w344:refnum<class "RemoteControl.STM.lvclass">, "Instrument"=w348:refnum<class "Instrument.lvclass">)
            n115 = call-dynamic "Read Configuration.vi"("error in (no error)"=w341, "Instrument in"=w348) -> ("error out"=w347:errorcluster, "Configuration"=w349:T11)  [unwired: 7 in, 1 out]
            n116 = Unbundle By Name(w349) -> ("SMO.VI Address"=w345:string, "SMO.Port"=w346:i32)
            n117 = call-dynamic "Open Client Connection.vi"("error in (no error)"=w347, "Port"=w346, "address"=w345, "RemoteControl.STM in"=w344) -> ("error out"=w340:errorcluster, "RemoteControl.STM out"=w339:refnum<class "RemoteControl.STM.lvclass">)  [unwired: 6 in]
            n118 = Bundle By Name(cluster=w343, "RC.STM"=w339) -> (w342:T7)
            n119 = call <vilib>:"Add State(s) to Queue__jki_lib_state_machine.vi"("State(s) in (\"\")"=w352) -> ("States Out"=w351:string)  [unwired: 14 in]
          }
          frame "Action: RC Send" {
            n120 = Unbundle By Name(w366) -> ("Instrument"=w353:refnum<class "Instrument.lvclass">, "RC.STM"=w364:refnum<class "RemoteControl.STM.lvclass">, "config"=w363:variant)
            n121 = case shown="\"getAll\"" w355 {
              tunnel: [FALSE ("Wait for response?") TRUE ("Wait for response?")] -> w354
              frame Default {
              }
              frame "getAll" {
              }
            }
            n122 = call-dynamic "Send and Receive Message.vi"("Wait for response?"=w354, "error in (no error)"=w362, "Data"=w363, "Command"=w355, "RemoteControl in"=w364) -> ("error out"=w359:errorcluster, "Data out"=w360:variant, "Command out"=w361:string, "RemoteControl out"=w356:refnum<class "RemoteControl.STM.lvclass">)  [unwired: 3 in]
            n123 = case shown="\"getAll\"" w361 {
              tunnel: ["" "Action: Update Front Panel All"] -> w358
              tunnel: w360 -> [_ w378]
              tunnel: [variant ("Data") w378] -> w357
              frame Default {
              }
              frame "getAll" {
              }
            }
            n124 = disable-structure shown="Disabled" {
              disable-tunnel: w353 -> [w373 _]
              frame Disabled {
                n125 = To More Specific Class(target class=refnum<class "instrument.PPMS2.lvclass"> refnum ("instrument.PPMS2 out"), reference=w373) -> (specific class reference=w372:refnum<class "instrument.PPMS2.lvclass">, error out=w370:errorcluster)  [unwired: 1 in]
                n126 = call-dynamic "Set Temperature.vi"("error in (no error)"=w370, "instrument.PPMS2 in"=w372) -> ()  [unwired: 8 in, 2 out]
              }
              frame Enabled {
              }
            }
            n127 = Bundle By Name(cluster=w366, "RC.STM"=w356, "getAll"=w357) -> (w365:T7)
            n128 = call <vilib>:"Add State(s) to Queue__jki_lib_state_machine.vi"("State(s) in Front (\"\")"=w358, "State(s) in (\"\")"=w369) -> ("States Out"=w368:string)  [unwired: 13 in]
          }
          frame "Action: Config" {
            # "#todo\nthis is configured to call Instrument.MessageToProcess.vi\nBut you could open a connection through STM and this can be a\nremote UI that runs from any machine (no examples are provided here\nyet (2/4/2019))\ndid this...3/29/2019. this state should be unused now(?)"
            n129 = Unbundle By Name(w385) -> ("Instrument"=w384:refnum<class "Instrument.lvclass">, "config"=w382:variant)
            n130 = call <userlib>:"Instrument.MessageToProcess.vi"("error in (no error)"=w381, "Message.Data"=w382, "Message.Command"=w380, "Instrument"=w384) -> ("error out"=w383:errorcluster)  [unwired: 6 in, 1 out]
            n131 = call <vilib>:"Add State(s) to Queue__jki_lib_state_machine.vi"("State(s) in (\"\")"=w388) -> ("States Out"=w387:string)  [unwired: 14 in]
          }
        }
      }
    }
    frame Error {
    }
  }
  n132 = call-parent "Process.vi"("error in (no error)"=w8, "SMO.UI"=w7) -> ("error out"=w5:errorcluster, "SMO.UI out"=→"Example Instrument UI out":refnum<class "Instrument.PPMS2 UI.lvclass">)  [unwired: 8 in]
  n133 = Merge Errors(w5, w4) -> (→"error out":errorcluster)
